vi "Get Object Pointer.vi"(11 "Tree in":refnum<class "Tree.lvclass">) -> (1 "Object Pointer":i64, 2 "Assigned object pointer?":bool, 3 "Tree out":refnum<class "Tree.lvclass">)   [LabVIEW 2012, in "MDSplus.lvlib" / "Tree.lvclass"]
uses:
  <vilib>/MDSplus/Classes/Tree_Class/Tree.lvclass
  <vilib>/MDSplus/Classes/Tree_Class/Tree.lvclass/Tree.ctl
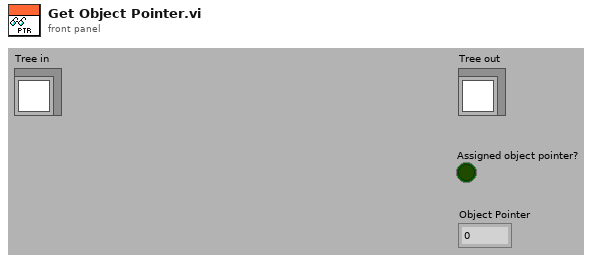
[diagram p1: front panel]
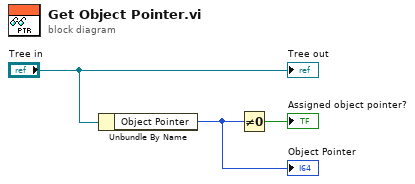
[diagram p0: block diagram]
diagram:
  n1 = Unbundle By Name("Tree in") -> ("Object Pointer"=w1:i64)
  "Object Pointer" <- w1
  n2 = Not Equal To 0?(x=w1) -> (x != 0?=→"Assigned object pointer?":bool)
  "Tree out" <- "Tree in"
